vi "gay.vi"() -> ()   [LabVIEW 2018]
panel:
  out "error out":errorcluster
  in  "error in (no error)":errorcluster
  in  "stop":bool
  in  "Y":dbl format="%#_13g"
  in  "X":dbl format="%#_13g"
  out "x+y":dbl[](array[numeric])
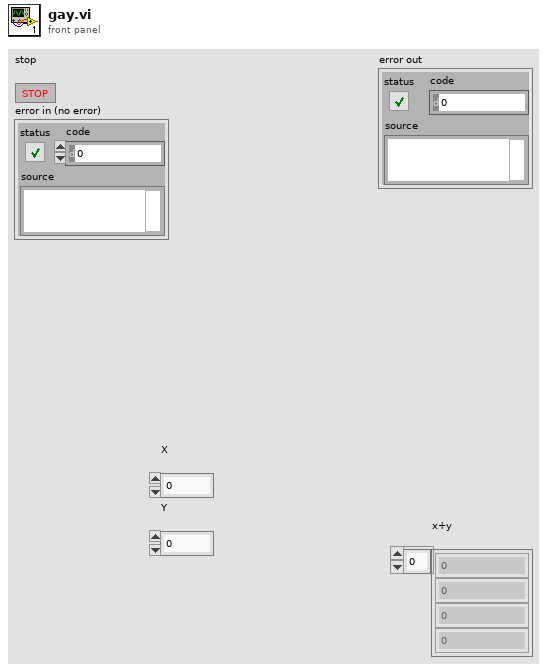
[diagram p1: front panel]
types:
  T1 = cluster{"proportional gain (Kc)":dbl, "integral time (Ti, min)":dbl, "derivative time (Td, min)":dbl}
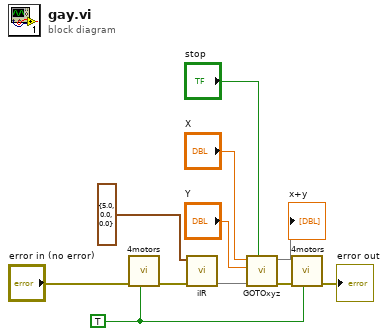
[diagram p0: block diagram]
diagram:
  w10 = TRUE ("Reset")
  n1 = call "4motors.vi"("Reset"=w10, "error in (no error)"="error in (no error)") -> ("error out"=w3:errorcluster)  [unwired: 8 in, 1 out]
  n2 = call "iIR.vi"(8:w3, "PID gains"=T1 {"proportional gain (Kc)"=5.0, "integral time (Ti, min)"=0.0, "derivative time (Td, min)"=0.0}) -> (0:w2)  [unwired: 7 in, 2 out]
  n3 = call "GOTOxyz.vi"("reset"="stop", "error in (no error)"=w2, "Y"="Y", "X"="X") -> ("error out"=w1:errorcluster, 3:→"x+y")  [unwired: 5 in]
  n4 = call "4motors.vi"("Reset"=w10, "error in (no error)"=w1) -> ("error out"=→"error out":errorcluster)  [unwired: 8 in, 1 out]
